vi "CLD 8 CSV file commands utility Solution.vi"(8 "Error In":errorcluster) -> (0 "Error Out":errorcluster, 3 "Commands Out Array":T1[](array[typedef]))   [LabVIEW 2020]
doc: "CLD 8: Reads data from CSV and inserts into array of clusters."
uses:
  CLD 8 Data Cluster.ctl
  <vilib>/Utility/file.llb/Read Delimited Spreadsheet (string).vi
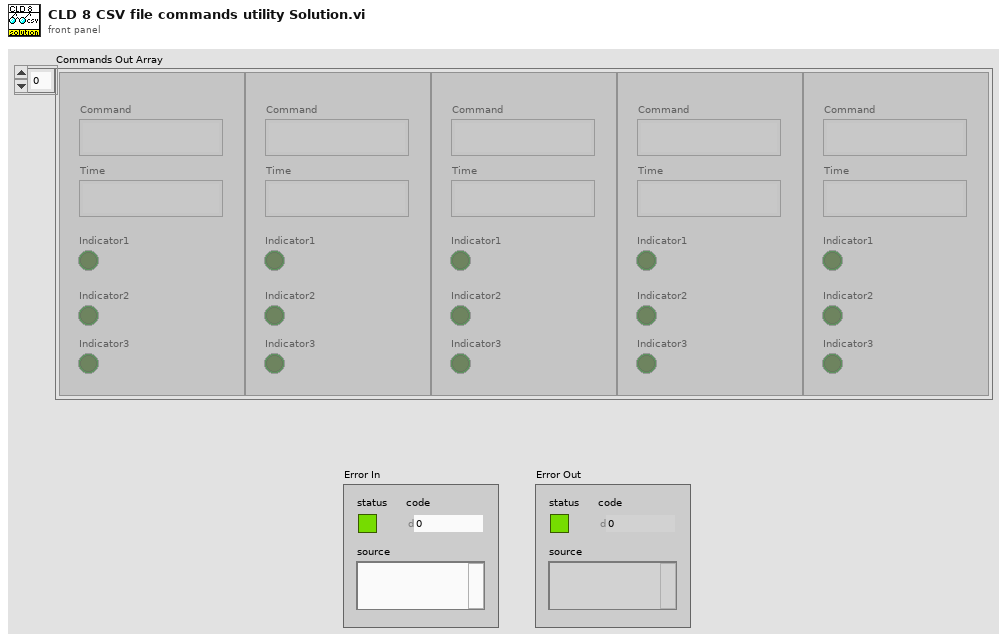
[diagram p1: front panel]
types:
  T1 = typedef "CLD 8 Data Cluster.ctl" = cluster{"Command":string, "Time":string, "Indicator1":bool, "Indicator2":bool, "Indicator3":bool}
  T2 = cluster{"[0]":bool, "[1]":bool, "[2]":bool, "[3]":bool, "[4]":bool, "[5]":bool, "[6]":bool, "[7]":bool, "[8]":bool}
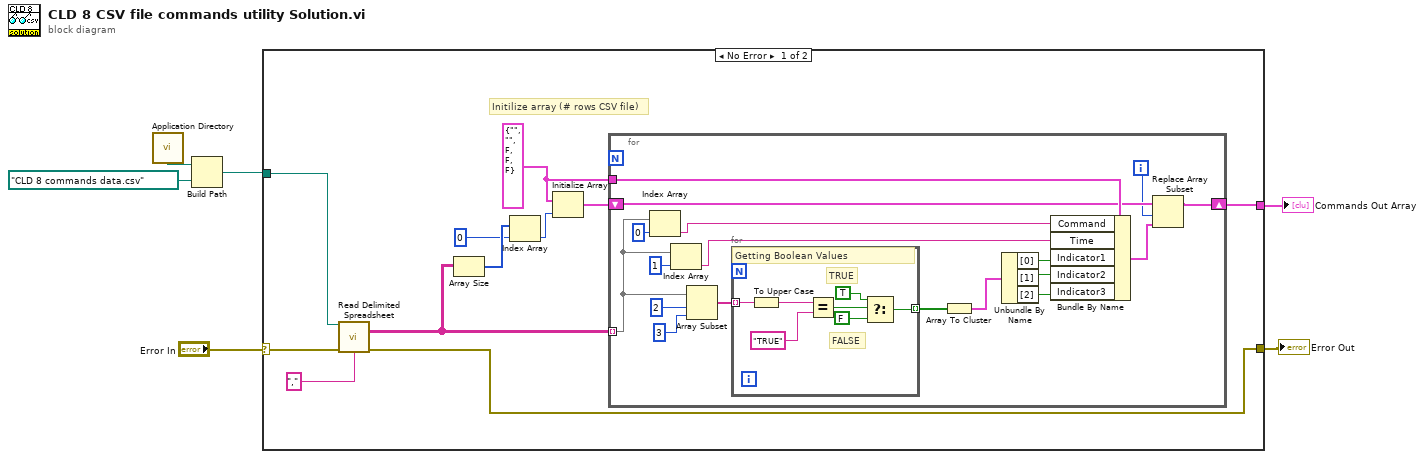
[diagram p0: block diagram]
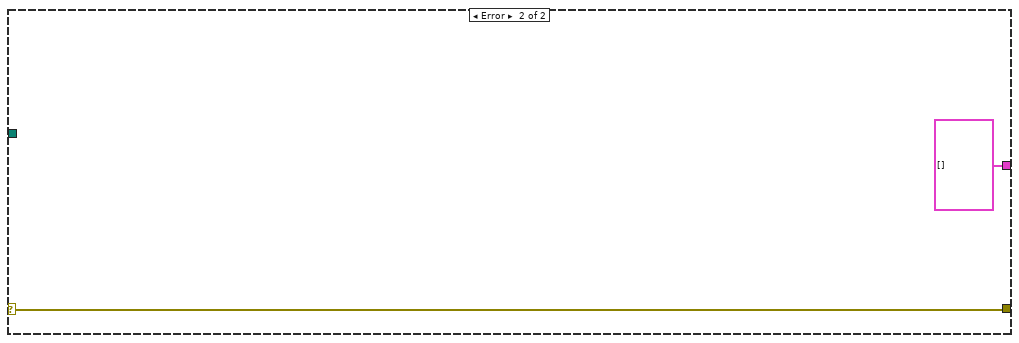
[diagram p2: hidden frame]
diagram:
  n1 = call <vilib>:"Application Directory.vi"() -> ("Application Directory"=w3:path)
  n2 = Build Path(base path=w3, name or relative path=path "CLD 8 commands data.csv") -> (appended path=w2:path)
  n3 = case shown="No Error" "Error In" {
    selector: "Error In" -> [w16 w44]
    tunnel: [w11 w44] -> w5
    tunnel: w2 -> [w17 _]
    tunnel: [w7 T1[] []] -> w1
    frame No Error {
      w8 = T1 {"Command"="", "Time"="", "Indicator1"=FALSE, "Indicator2"=FALSE, "Indicator3"=FALSE} ("Cluster")
      # "Initilize array (# rows CSV file)"
      n4 = call-poly <vilib>:"Read Delimited Spreadsheet.vi"("file path (dialog if empty)"=w17, "error in (no error)"=w16, "delimiter (\\t)"="," ("delimiter (\\t)")) -> ("all rows"=w10:string[][], "error out"=w11:errorcluster)  [unwired: 7 in, 4 out]
      n5 = Array Size(array=w10) -> (size(s)=w14:i32[])
      n6 = Index Array(array=w14, index=0) -> (element=w12:i32)
      n7 = Initialize Array(w8, w12) -> (w9:T1[])
      n8 = for {
        tunnel: w10 -> [w26] mode=indexing
        shift-right: [w34] -> w7
        shift-left: w9 -> [w33]
        tunnel: w8 -> [w35]
        i -> [w31]
        n9 = Index Array(array=w26, index=0) -> (element=w30:string)
        n10 = Index Array(array=w26, index=1) -> (element=w28:string)
        n11 = Array Subset(array=w26, index=2, length=3) -> (w23:string[])
        n12 = for {
          tunnel: w23 -> [w41] mode=indexing
          tunnel: [w36] -> w22 mode=indexing
          # "FALSE"
          # "TRUE"
          # "Getting Boolean Values"
          n13 = To Upper Case(1:w41) -> (0:w40:string)
          n14 = Equal?(x=w40, y="TRUE") -> (x = y?=w38:bool)
          n15 = Select(t=TRUE, s=w38, f=FALSE) -> (s? t:f=w36:bool)
        }
        n16 = Array To Cluster(array=w22) -> (cluster=w21:T2)
        n17 = Unbundle By Name(w21) -> ("[0]"=w20:bool, "[1]"=w19:bool, "[2]"=w18:bool)
        n18 = Bundle By Name(cluster=w35, "Command"=w30, "Time"=w28, "Indicator1"=w20, "Indicator2"=w19, "Indicator3"=w18) -> (w32:T1)
        n19 = Replace Array Subset(array=w33, new element=w32, index=w31) -> (w34:T1[])
      }
    }
    frame Error {
    }
  }
  "Error Out" <- w5
  "Commands Out Array" <- w1
